vi "Define Mask.vi"(8 "error in (no error)":errorcluster, 11 "FPGA Image":T3(plugin-control)=refnum) -> (0 "error out":errorcluster)   [LabVIEW 2013]
doc: "GUI for selecting a part type and starting a batch process\nPart types list is passed in from caller.\nReturns when Start or Cancel is pressed."
uses:
  Sectors/Number of Wing Sector.ctl
  Mask ROI FG Enum.ctl
  Mask ROI Cluster.ctl
  Common/File IO/INI/Read write mode.ctl
  Message Passing/MsgQ Loops enum.ctl
  System Status/Status FG Enum.ctl
  Common/State Machines/State Machine Lib.lvlib
  Common/GUI/GUI.lvlib
  <vilib>/vision/NI_Vision_Development_Module.lvlib
  Image Processing.lvlib
  Message Passing/Main MsgQ.lvlib
panel:
  in  "Calculate BG":bool
  in  "Load Current Mask":bool
  out "Right ROI":T1 {"Contours"."Type" items=["No Selection", "Point", "Line", "Rectangle", "Oval", "Polygon", "Freehand Region", "Annulus", "Unused2", "Unused3", "Broken Line", "Freehand Line", "Rotated Rectangle"]}
  out "Left ROI":T1 {"Contours"."Type" items=["No Selection", "Point", "Line", "Rectangle", "Oval", "Polygon", "Freehand Region", "Annulus", "Unused2", "Unused3", "Broken Line", "Freehand Line", "Rotated Rectangle"]}
  out "[Avg BG]":dbl[](array[numeric])
  in  "NumWingSectors":T2=1 items=["1"=1, "2"=2, "4"=4, "8"=8, "16"=16]
  out "State":string
  in  "Exit":bool
  in  "Save Mask":bool
  out "combo mask":T3(plugin-control)
  out "right mask":T3(plugin-control)
  out "right masked image":T3(plugin-control)
  out "right annulus":T4={"Center X"=929, "Center Y"=663, "Inner Radius"=200, "Outer Radius"=405, "Start Angle"=90.0, "End Angle"=180.0} {"End Angle" format="%.2f"; "Start Angle" format="%.2f"; "Center X" scale=0.0..1024.0}
  out "left mask":T3(plugin-control)
  out "left masked image":T3(plugin-control)
  out "left annulus":T4={"Center X"=929, "Center Y"=663, "Inner Radius"=200, "Outer Radius"=405, "Start Angle"=90.0, "End Angle"=180.0} {"End Angle" format="%.2f"; "Start Angle" format="%.2f"; "Center X" scale=0.0..1024.0}
  in  "Accept Threshold":bool
  out "Processed Image":T3(plugin-control)
  in  "Threshold Range":cluster{"Lower value":dbl, "Upper value":dbl}={"Lower value"=106.82432432432432, "Upper value"=255.0} {"Upper value" min=0.0 max=255.0 scale=0.0..255.0; "Lower value" min=0.0 max=255.0}
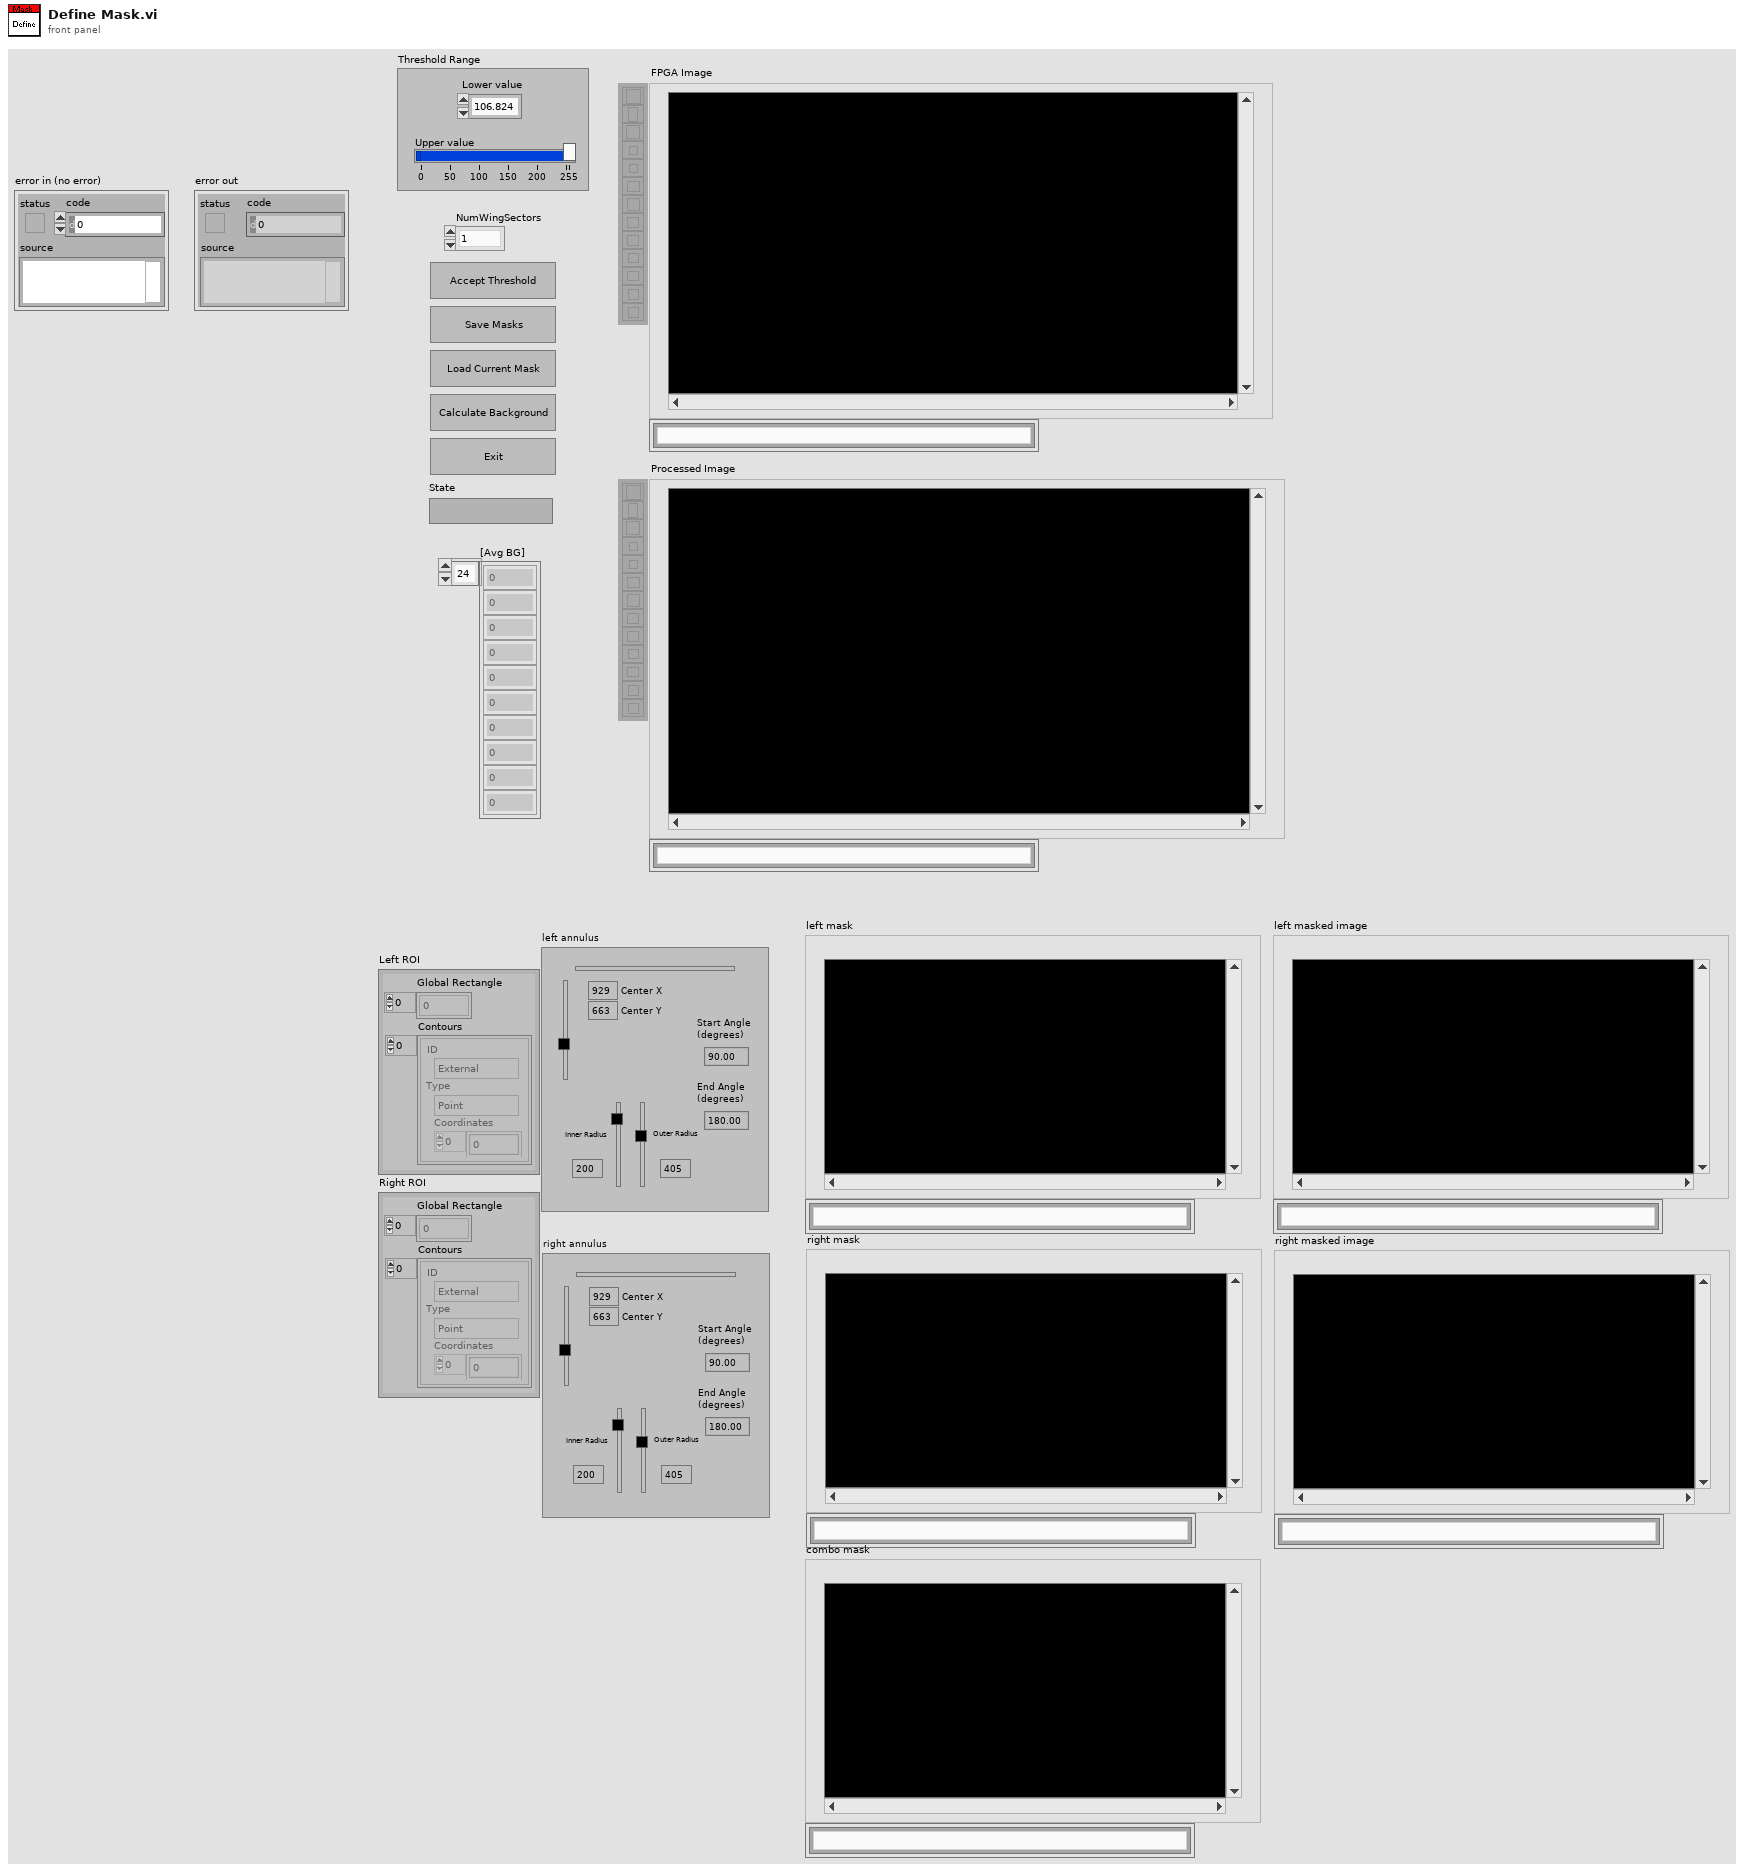
[diagram p1: front panel]
types:
  T1 = typedef "ROI Descriptor" = cluster{"Global Rectangle":i32[], "Contours":cluster{"ID":enum32{"External", "Internal"}, "Type":u32, "Coordinates":i32[]}[]}
  T2 = typedef "Number of Wing Sector.ctl" = u8
  T3 = typedef "IMAQ Image.ctl" = refnum<image>
  T4 = typedef "IMAQ Circle" = cluster{"Center X":i32, "Center Y":i32, "Inner Radius":i32, "Outer Radius":i32, "Start Angle":dbl, "End Angle":dbl}
  T5 = typedef "State Machine Lib.lvlib/STATE cluster.ctl" = cluster{"State":string, "Parameters":variant}
  T6 = typedef "Mask ROI FG Enum.ctl" = enum16{"Read", "Write", "Enable Background", "Disable Background"}
  T7 = typedef "Main MsgQ.lvlib/MsgQ Loops enum.ctl" = enum16{"User Interface", "Image Acq"}
  T8 = typedef "Read write mode.ctl" = enum16{"Read", "Write"}
  T9 = typedef "Mask ROI Cluster.ctl" = cluster{"left annulus":T4, "right annulus":T4, "Threshold Range":cluster{"Lower value":dbl, "Upper value":dbl}, "[Avg BG]":u8[], "Number of Sectors":u8, "Left ROI":T1, "Right ROI":T1, "Left Start Angle Duty Cycle":fxp<+,8,0>, "Left End Angle Duty Cycle":fxp<+,8,0>, "Right End Angle Duty Cycle":fxp<+,8,0>, "Right Start Angle Duty Cycle":fxp<+,8,0>, "[Sector ROIs]":T1[]}
  T10 = typedef "Status FG Enum.ctl" = enum16{"Reset", "Read", "Write"}
  T11 = typedef "Sector Parameter Cluster.ctl" = cluster{"Start Angle":fxp<+/-,17,2>, "End Angle":fxp<+/-,17,2>, "Inner Radius":u16, "Outter Radius":u16, "Hinge X":u16, "Hinge Y":u16, "NumWingSectors":u8}
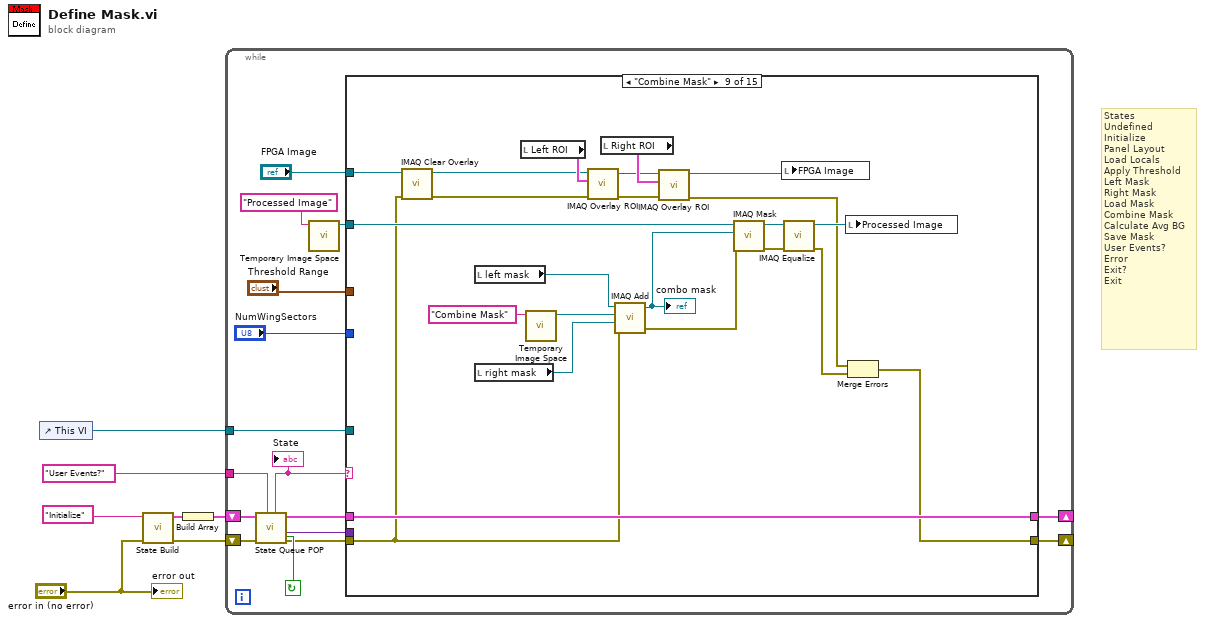
[diagram p0: block diagram]
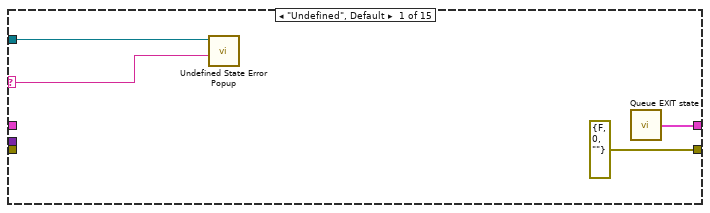
[diagram p2: hidden frame]
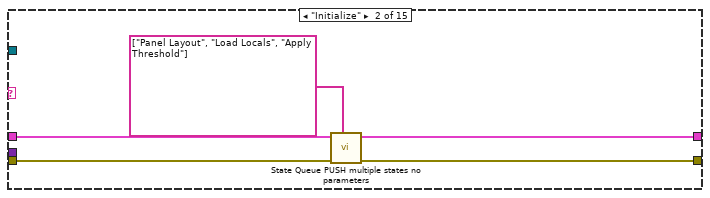
[diagram p3: hidden frame]
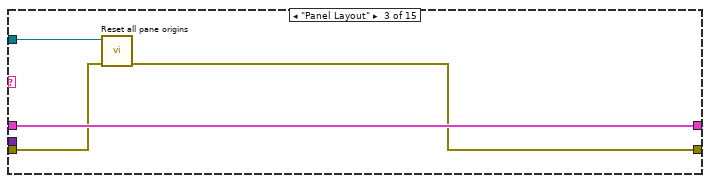
[diagram p4: hidden frame]
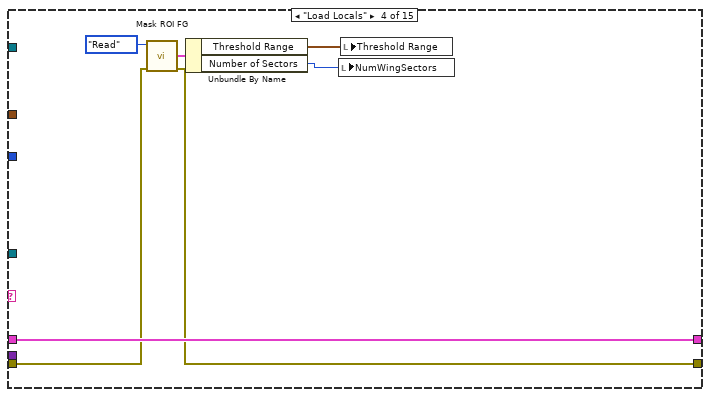
[diagram p5: hidden frame]
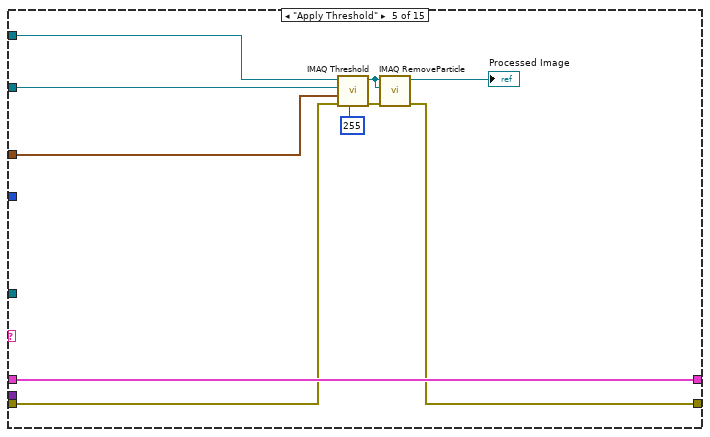
[diagram p6: hidden frame]
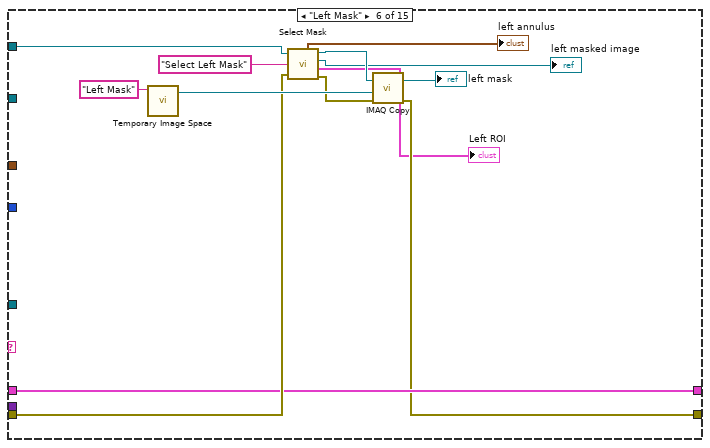
[diagram p7: hidden frame]
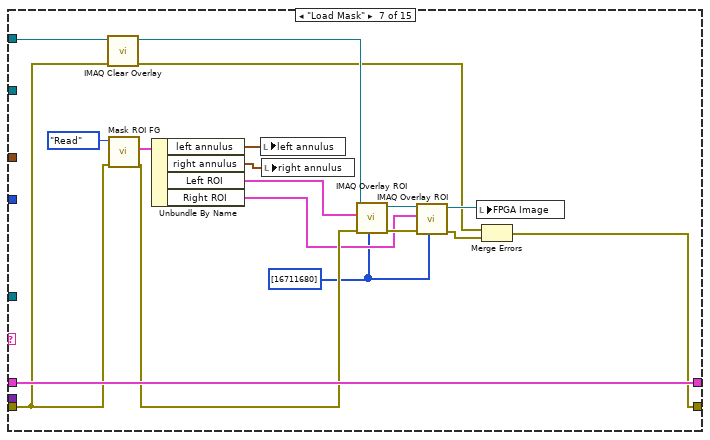
[diagram p8: hidden frame]
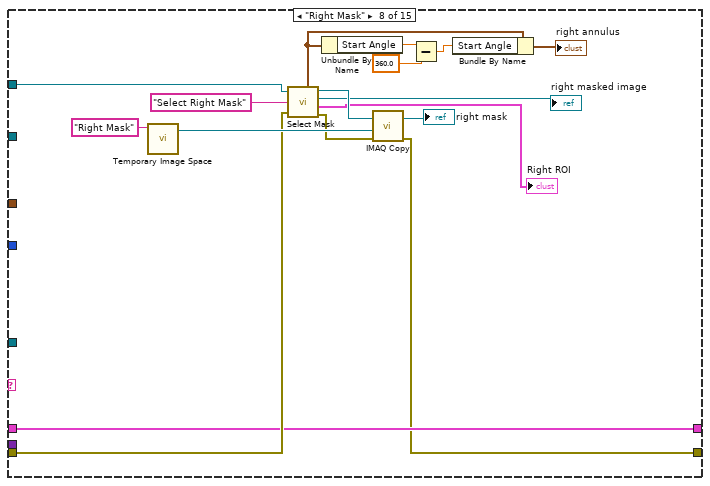
[diagram p9: hidden frame]
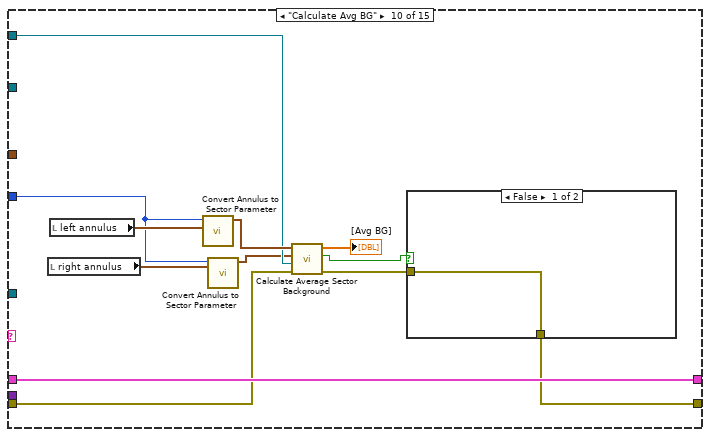
[diagram p10: hidden frame]
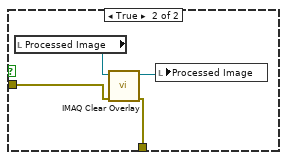
[diagram p11: hidden frame]
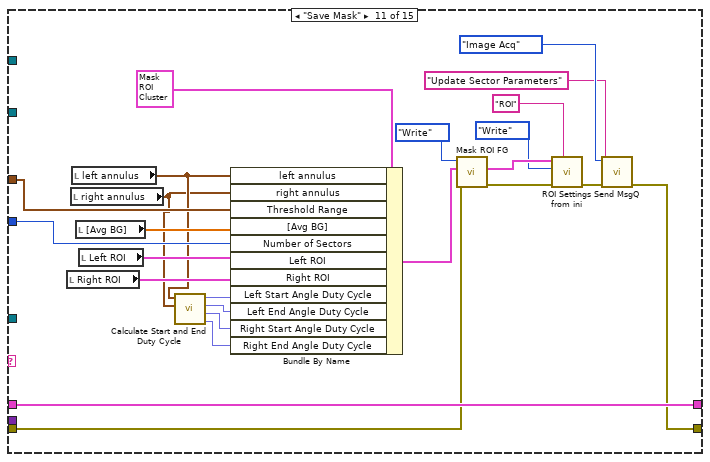
[diagram p12: hidden frame]
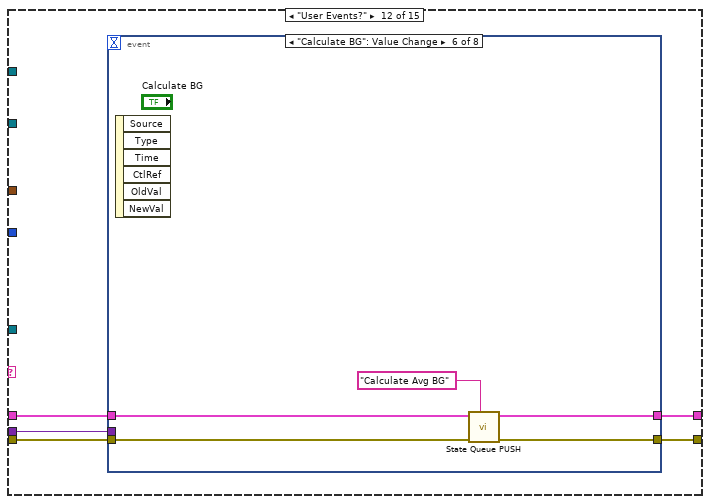
[diagram p13: hidden frame]
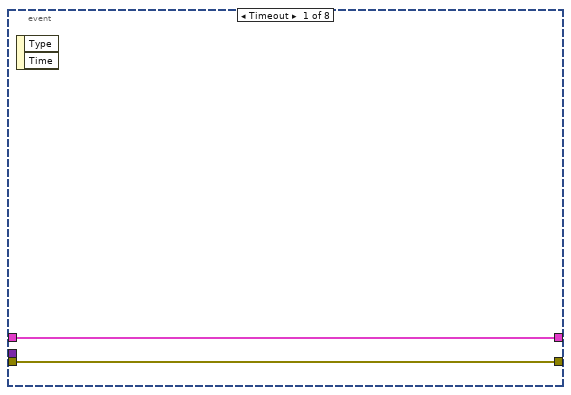
[diagram p14: hidden frame]
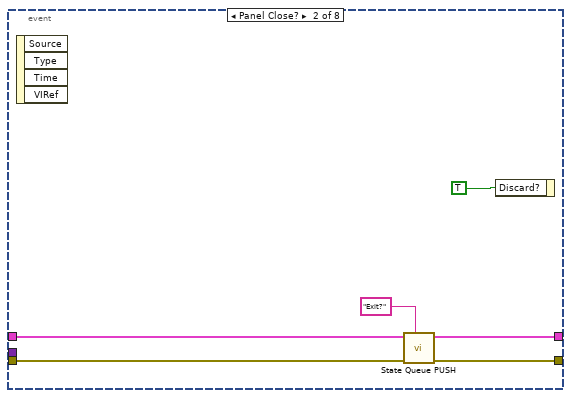
[diagram p15: hidden frame]
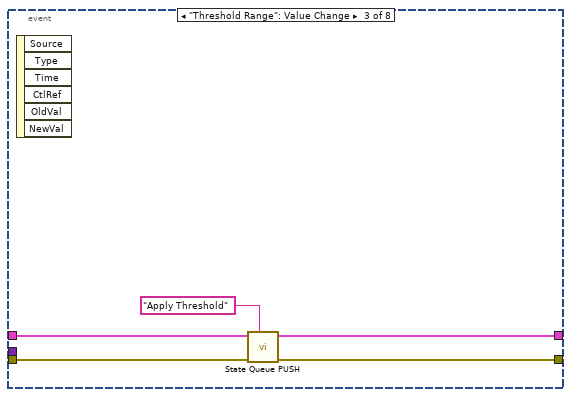
[diagram p16: hidden frame]
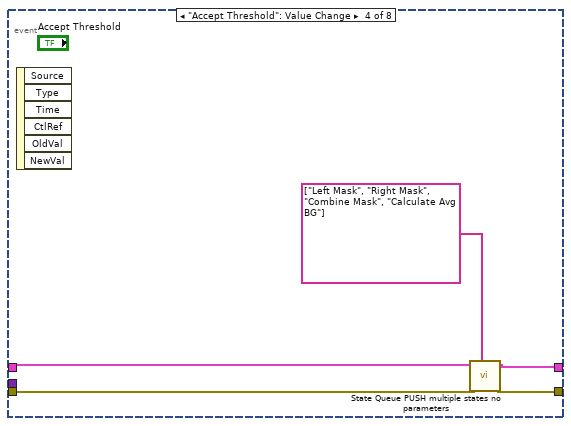
[diagram p17: hidden frame]
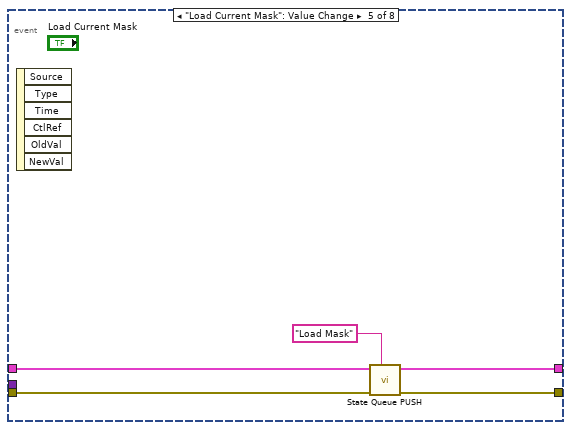
[diagram p18: hidden frame]
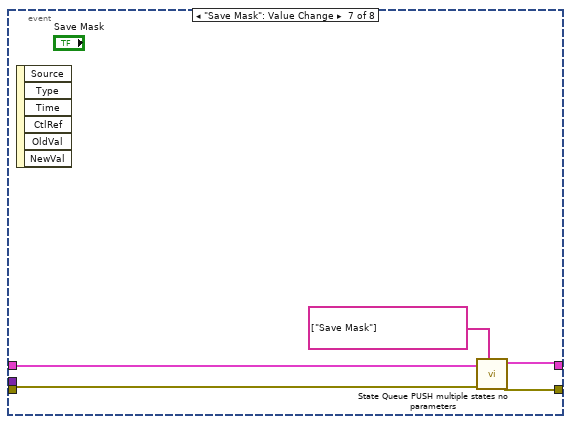
[diagram p19: hidden frame]
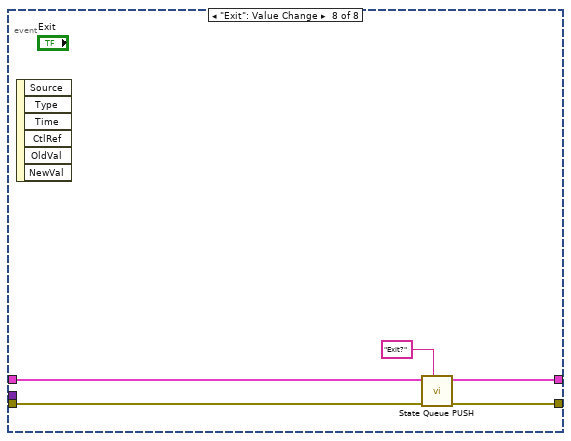
[diagram p20: hidden frame]
diagram:
  # "States\nUndefined\nInitialize\nPanel Layout\nLoad Locals\nApply Threshold\nLeft Mask\nRight Mask\nLoad Mask\nCombine Mask\nCalculate Avg BG\nSave Mask\nUser Events?\nError\nExit?\nExit"
  n1 = control-ref of="This VI"() -> (w6:refnum<vi>)
  n2 = call "State Build.vi"("error in (no error)"="error in (no error)", "State"="Initialize") -> ("error out"=w3:errorcluster, "State Out"=w4:T5)  [unwired: 8 in]
  n3 = Build Array(w4) -> (w5:T5[])
  n4 = while {
    shift-right: [w14] -> _
    shift-left: w3 -> [w22]
    shift-right: [w13] -> _
    shift-left: w5 -> [w20]
    tunnel: "User Events?" ("Default state") -> [w21]
    tunnel: w6 -> [w16]
    stop <- w23 continue-if-true
    n5 = call "State Queue POP.vi"("Default state"=w21, "error in (no error)"=w22, "State que in"=w20) -> ("error out"=w19:errorcluster, "Parameters"=w15:variant, "State que out"=w18:T5[], "Not Exit?"=w23:bool, "State case out"=w17:string)  [unwired: 4 out]
    "State" <- w17
    n6 = call "Temporary Image Space.vi"("Image Name"="Processed Image") -> ("Image Out"=w10:T3)  [unwired: 10 in]
    n7 = case shown="\"Combine Mask\"" w17 {
      selector: w17 -> [w24 _ _ _ _ _ _ _ _ _ _ _ _ _ _]
      tunnel: w19 -> [_ w30 w34 w42 w48 w59 w72 w94 w109 w135 w160 w169 w209 w223 w226]
      tunnel: w18 -> [_ w32 w36 w43 w49 w58 w83 w93 w114 w136 w165 w170 _ w217 w228]
      tunnel: w16 -> [w25 _ w35 _ _ _ _ _ _ _ _ _ _ _ _]
      tunnel: w15 -> [_ _ _ _ _ _ _ _ _ _ _ w168 _ _ _]
      tunnel: [errorcluster {"status"=FALSE, "code"=0, "source"=""} ("error out") w31 w33 w37 w47 w57 w67 w92 w102 w126 w150 w167 errorcluster {"status"=FALSE, "code"=0, "source"=""} ("error out") w223 w224] -> w14
      tunnel: [w27 w28 w36 w43 w49 w58 w83 w93 w114 w136 w165 w166 w214 w216 w228] -> w13
      tunnel: "Threshold Range" -> [_ _ _ _ w46 _ _ _ _ _ w162 _ _ _ _]
      tunnel: "FPGA Image" -> [_ _ _ _ w45 w60 w73 w95 w110 w132 _ _ _ _ w227]
      tunnel: w10 -> [_ _ _ _ w44 _ _ _ w117 _ _ _ _ _ _]
      tunnel: "NumWingSectors" -> [_ _ _ _ _ _ _ _ _ w130 w158 _ _ _ _]
      frame "Undefined", Default {
        n8 = call "Undefined State Error Popup.vi"("String"=w24, "This VI (Caller if unwired)"=w25) -> ()  [unwired: 10 out]
        n9 = call "Queue EXIT state.vi"() -> ("Exit State Q"=w27:T5[])  [unwired: 1 in]
      }
      frame "Initialize" {
        n10 = call "State Queue PUSH multiple states no parameters.vi"("States to queue"=string[] ["Panel Layout", "Load Locals", "Apply Threshold"], "error in (no error)"=w30, "State que in"=w32) -> ("error out"=w31:errorcluster, "State que out"=w28:T5[])  [unwired: 1 in, 6 out]
      }
      frame "Panel Layout" {
        n11 = call "Reset all pane origins.vi"("error in (no error"=w34, "Vi Ref In"=w35) -> ("error out"=w33:errorcluster)  [unwired: 9 out]
      }
      frame "Load Locals" {
        n12 = call "Mask ROI FG.vi"("error in (no error)"=w42, "Operation"=Mask_ROI_FG_Enum."Read") -> ("error out"=w37:errorcluster, "Mask ROI Out"=w40:T9)  [unwired: 8 in]
        n13 = Unbundle By Name(w40) -> ("Threshold Range"=w39:cluster{"Lower value":dbl, "Upper value":dbl}, "Number of Sectors"=w38:u8)
        n14 = local write "NumWingSectors"(w38) -> ()
        n15 = local write "Threshold Range"(w39) -> ()
      }
      frame "Apply Threshold" {
        n16 = call "IMAQ Threshold"("Replace Value"=u8 255, "error in (no error)"=w48, "Range"=w46, "Image Dst"=w44, "Image Src"=w45) -> ("error out"=w51:errorcluster, "Image Dst Out"=w53:T3)  [unwired: 1 in, 4 out]
        n17 = call "IMAQ RemoveParticle"("error in (no error)"=w51, "Image Dst"=w53, "Image Src"=w53) -> ("error out"=w47:errorcluster, "Image Dst Out"=→"Processed Image":T3)  [unwired: 4 in, 3 out]
      }
      frame "Left Mask" {
        n18 = call "Temporary Image Space.vi"("Image Name"="Left Mask") -> ("Image Out"=w61:T3)  [unwired: 10 in]
        n19 = call "Select Mask.vi"("error in"=w59, "Prompt"="Select Left Mask", "Read \nImage"=w60) -> ("error out"=w56:errorcluster, "ROI Descriptor Out"=→"Left ROI":T1, "Masked \nImage"=→"left masked image":T3, "Annulus"=→"left annulus":T4, "mask"=w64:T3)  [unwired: 1 out]
        n20 = call "IMAQ Copy"("error in (no error)"=w56, "Image Dst"=w61, "Image Src"=w64) -> ("error out"=w57:errorcluster, "Image Dst Out"=→"left mask":T3)  [unwired: 3 in]
      }
      frame "Load Mask" {
        w70 = u32[] [16711680] ("Colors (Green)")
        n21 = call "IMAQ Clear Overlay"("error in (no error)"=w72, "Image"=w73) -> ("error out"=w69:errorcluster, "Image Out"=w71:T3)  [unwired: 8 in]
        n22 = call "Mask ROI FG.vi"("error in (no error)"=w72, "Operation"=Mask_ROI_FG_Enum."Read") -> ("error out"=w76:errorcluster, "Mask ROI Out"=w82:T9)  [unwired: 8 in]
        n23 = Unbundle By Name(w82) -> ("left annulus"=w81:T4, "right annulus"=w80:T4, "Left ROI"=w75:T1, "Right ROI"=w74:T1)
        n24 = local write "left annulus"(w81) -> ()
        n25 = local write "right annulus"(w80) -> ()
        n26 = call "IMAQ Overlay ROI"("Colors (Green)"=w70, "error in (no error)"=w76, "ROI Descriptor"=w75, "Image"=w71) -> ("error out"=w77:errorcluster, "Image Out"=w79:T3)  [unwired: 6 in]
        n27 = call "IMAQ Overlay ROI"("Colors (Green)"=w70, "error in (no error)"=w77, "ROI Descriptor"=w74, "Image"=w79) -> ("error out"=w68:errorcluster, "Image Out"=w78:T3)  [unwired: 6 in]
        n28 = local write "FPGA Image"(w78) -> ()
        n29 = Merge Errors(w69, w68) -> (w67:errorcluster)
      }
      frame "Right Mask" {
        n30 = call "Temporary Image Space.vi"("Image Name"="Right Mask") -> ("Image Out"=w96:T3)  [unwired: 10 in]
        n31 = call "Select Mask.vi"("error in"=w94, "Prompt"="Select Right Mask", "Read \nImage"=w95) -> ("error out"=w91:errorcluster, "ROI Descriptor Out"=→"Right ROI":T1, "Masked \nImage"=→"right masked image":T3, "Annulus"=w85:T4, "mask"=w99:T3)  [unwired: 1 out]
        n32 = Unbundle By Name(w85) -> ("Start Angle"=w90:dbl)
        n33 = call "IMAQ Copy"("error in (no error)"=w91, "Image Dst"=w96, "Image Src"=w99) -> ("error out"=w92:errorcluster, "Image Dst Out"=→"right mask":T3)  [unwired: 3 in]
        n34 = Subtract(x=w90, y=360.0) -> (x-y=w88:dbl)
        n35 = Bundle By Name(cluster=w85, "Start Angle"=w88) -> (→"right annulus":T4)
      }
      frame "Combine Mask" {
        n36 = call "IMAQ Clear Overlay"("error in (no error)"=w109, "Image"=w110) -> ("error out"=w108:errorcluster, "Image Out"=w107:T3)  [unwired: 8 in]
        n37 = local read "left mask"() -> (w119:T3)
        n38 = local read "right mask"() -> (w118:T3)
        n39 = local read "Left ROI"() -> (w113:T1)
        n40 = call "Temporary Image Space.vi"("Image Name"="Combine Mask") -> ("Image Out"=w121:T3)  [unwired: 10 in]
        n41 = call "IMAQ Overlay ROI"("error in (no error)"=w108, "ROI Descriptor"=w113, "Image"=w107) -> ("error out"=w106:errorcluster, "Image Out"=w105:T3)  [unwired: 7 in]
        n42 = local read "Right ROI"() -> (w112:T1)
        n43 = call "IMAQ Add"("Image Src A"=w119, "Image Dst"=w121, "Image Src B"=w118, "error in (no error)"=w109) -> ("Image Dst Out"=w122:T3, "error out"=w115:errorcluster)  [unwired: 3 in]
        "combo mask" <- w122
        n44 = call "IMAQ Overlay ROI"("error in (no error)"=w106, "ROI Descriptor"=w112, "Image"=w105) -> ("error out"=w104:errorcluster, "Image Out"=w111:T3)  [unwired: 7 in]
        n45 = call "IMAQ Mask"("error in (no error)"=w115, "Image Mask"=w122, "Image Src"=w117) -> ("error out"=w123:errorcluster, "Image Dst Out"=w124:T3)  [unwired: 1 in, 1 out]
        n46 = local write "FPGA Image"(w111) -> ()
        n47 = call "IMAQ Equalize"("error in (no error)"=w123, "Image Src"=w124) -> ("error out"=w103:errorcluster, "Image Dst Out"=w116:T3)  [unwired: 4 in, 4 out]
        n48 = local write "Processed Image"(w116) -> ()
        n49 = Merge Errors(w104, w103) -> (w102:errorcluster)
      }
      frame "Calculate Avg BG" {
        n50 = local read "right annulus"() -> (w129:T4)
        n51 = local read "left annulus"() -> (w134:T4)
        n52 = call "Convert Annulus to Sector Parameter.vi"("Annulus"=w134, "NumWingSectors"=w130) -> ("Sector Parameter"=w133:T11)  [unwired: 9 in]
        n53 = call "Convert Annulus to Sector Parameter.vi"("Annulus"=w129, "NumWingSectors"=w130) -> ("Sector Parameter"=w128:T11)  [unwired: 9 in]
        n54 = call "Calculate Average Sector Background.vi"("error in (no error)"=w135, "Image"=w132, "Right Sector Parameters"=w128, "Left Sector Parameters"=w133) -> ("error out"=w127:errorcluster, "Canceled?"=w125:bool, "[Avg BG]"=→"[Avg BG]":dbl[])  [unwired: 5 in]
        n55 = case shown="False" w125 {
          tunnel: w127 -> [w137 w140]
          tunnel: [w137 w139] -> w126
          frame False {
          }
          frame True {
            n56 = local read "Processed Image"() -> (w141:T3)
            n57 = call "IMAQ Clear Overlay"("error in (no error)"=w140, "Image"=w141) -> ("error out"=w139:errorcluster, "Image Out"=w138:T3)  [unwired: 8 in]
            n58 = local write "Processed Image"(w138) -> ()
          }
        }
      }
      frame "Save Mask" {
        n59 = local read "Right ROI"() -> (w148:T1)
        n60 = local read "right annulus"() -> (w146:T4)
        n61 = local read "left annulus"() -> (w147:T4)
        n62 = local read "[Avg BG]"() -> (w159:dbl[])
        n63 = local read "Left ROI"() -> (w149:T1)
        n64 = call "Calculate Start and End Duty Cycle.vi"("right annulus"=w146, "left annulus"=w147) -> ("Right End Angle Duty Cycle"=w142:fxp<+,8,0>, "Right Start Angle Duty Cycle"=w143:fxp<+,8,0>, "Left End Angle Duty Cycle"=w144:fxp<+,8,0>, "Left Start Angle Duty Cycle"=w145:fxp<+,8,0>)  [unwired: 6 in]
        n65 = Bundle By Name(cluster=T9 {"left annulus"={"Center X"=929, "Center Y"=663, "Inner Radius"=200, "Outer Radius"=405, "Start Angle"=90.0, "End Angle"=180.0}, "right annulus"={"Center X"=929, "Center Y"=663, "Inner Radius"=200, "Outer Radius"=405, "Start Angle"=90.0, "End Angle"=180.0}, "Threshold Range"={"Lower value"=106.82432432432432, "Upper value"=255.0}, "[Avg BG]"=[], "Number of Sectors"=0, "Left ROI"={"Global Rectangle"=[], "Contours"=[]}, "Right ROI"={"Global Rectangle"=[], "Contours"=[]}, "Left Start Angle Duty Cycle"=0.0, "Left End Angle Duty Cycle"=0.0, "Right End Angle Duty Cycle"=0.0, "Right Start Angle Duty Cycle"=0.0, "[Sector ROIs]"=[]} ("Mask ROI In"), "left annulus"=w147, "right annulus"=w146, "Threshold Range"=w162, "[Avg BG]"=w159, "Number of Sectors"=w158, "Left ROI"=w149, "Right ROI"=w148, "Left Start Angle Duty Cycle"=w145, "Left End Angle Duty Cycle"=w144, "Right Start Angle Duty Cycle"=w143, "Right End Angle Duty Cycle"=w142) -> (w161:T9)
        n66 = call "Mask ROI FG.vi"("error in (no error)"=w160, "Mask ROI In"=w161, "Operation"=Mask_ROI_FG_Enum."Write") -> ("error out"=w155:errorcluster, "Mask ROI Out"=w157:T9)  [unwired: 7 in]
        n67 = call "ROI Settings from ini.vi"("Section"="ROI", "error in (no error)"=w155, "Operation"=Read_write_mode."Write", "Mask ROI In"=w157) -> ("error out"=w151:errorcluster)  [unwired: 5 in, 2 out]
        n68 = call "Send MsgQ.vi"("error in (no error)"=w151, "Message String"="Update Sector Parameters", "Send to MsgQ"=MsgQ_Loops_enum."Image Acq") -> ("error out"=w150:errorcluster)  [unwired: 8 in]
      }
      frame "User Events?" {
        n69 = event shown="[5] \"Calculate BG\": Value Change" {
          selector: _ -> [_ _ _ _ _ _ _ _]
          dyn-events: _ -> [_ _ _ _ _ _ _ _]
          timeout: _ -> [_ _ _ _ _ _ _ _]
          tunnel: w170 -> [w171 w177 w183 w186 w192 w197 w202 w205]
          tunnel: w169 -> [w172 w176 w182 w184 w189 w194 w199 w206]
          tunnel: w168 -> [_ _ _ _ _ _ _ _]
          tunnel: [w172 w174 w180 w187 w190 w195 w200 w207] -> w167
          tunnel: [w171 w175 w181 w188 w191 w196 w201 w208] -> w166
          event Timeout {
            n70 = event-data() -> ()  [unwired: 3 out]
          }
          event Panel Close? {
            n71 = event-data() -> ()  [unwired: 5 out]
            n72 = call "State Queue PUSH.vi"("State case"="Exit?", "error in (no error)"=w176, "State que in"=w177) -> ("error out"=w174:errorcluster, "State que out"=w175:T5[])  [unwired: 2 in, 5 out]
            n73 = event-data("Discard?"=TRUE) -> ()  [unwired: 1 in, 1 out]
          }
          event "Threshold Range": Value Change {
            n74 = event-data() -> ()  [unwired: 7 out]
            n75 = call "State Queue PUSH.vi"("State case"="Apply Threshold", "error in (no error)"=w182, "State que in"=w183) -> ("error out"=w180:errorcluster, "State que out"=w181:T5[])  [unwired: 2 in, 5 out]
          }
          event "Accept Threshold": Value Change {
            n76 = event-data() -> ()  [unwired: 7 out]
            n77 = call "State Queue PUSH multiple states no parameters.vi"("States to queue"=string[] ["Left Mask", "Right Mask", "Combine Mask", "Calculate Avg BG"], "error in (no error)"=w184, "State que in"=w186) -> ("error out"=w187:errorcluster, "State que out"=w188:T5[])  [unwired: 7 in]
          }
          event "Load Current Mask": Value Change {
            n78 = event-data() -> ()  [unwired: 7 out]
            n79 = call "State Queue PUSH.vi"("State case"="Load Mask", "error in (no error)"=w189, "State que in"=w192) -> ("error out"=w190:errorcluster, "State que out"=w191:T5[])  [unwired: 2 in, 5 out]
          }
          event "Calculate BG": Value Change {
            n80 = event-data() -> ()  [unwired: 7 out]
            n81 = call "State Queue PUSH.vi"("State case"="Calculate Avg BG", "error in (no error)"=w194, "State que in"=w197) -> ("error out"=w195:errorcluster, "State que out"=w196:T5[])  [unwired: 2 in, 5 out]
          }
          event "Save Mask": Value Change {
            n82 = event-data() -> ()  [unwired: 7 out]
            n83 = call "State Queue PUSH multiple states no parameters.vi"("States to queue"=string[] ["Save Mask"], "error in (no error)"=w199, "State que in"=w202) -> ("error out"=w200:errorcluster, "State que out"=w201:T5[])  [unwired: 7 in]
          }
          event "Exit": Value Change {
            n84 = event-data() -> ()  [unwired: 7 out]
            n85 = call "State Queue PUSH.vi"("State case"="Exit?", "error in (no error)"=w206, "State que in"=w205) -> ("error out"=w207:errorcluster, "State que out"=w208:T5[])  [unwired: 7 in]
          }
        }
      }
      frame "Error" {
        # "DEFAULT IS \nTO CLEAR ERROR\nAND EXIT"
        n86 = Unbundle By Name(w209) -> ("source"=w212:string)
        n87 = Concatenate Strings("Error: " ("string"), w212) -> (w211:string)
        n88 = call "Status FG.vi"("Status In"=w211, "Operation"=Status_FG_Enum."Write") -> ()  [unwired: 8 in, 2 out]
        n89 = call <vilib>:"Clear Errors.vi"("error in (no error)"=w209) -> ()  [unwired: 7 out]
        n90 = call "Queue EXIT state.vi"() -> ("Exit State Q"=w214:T5[])  [unwired: 1 in]
      }
      frame "Exit?" {
        n91 = Two Button Dialog(message="Exit?", 1:"No" ("F button name (\"Cancel\")"), 2:"Yes" ("T button name (\"OK\")")) -> (T button?=w219:bool)
        n92 = call "Queue EXIT state.vi"() -> ("Exit State Q"=w218:T5[])  [unwired: 1 in]
        n93 = Select(t=w218, s=w219, f=w217) -> (s? t:f=w216:T5[])
      }
      frame "Exit" {
        n94 = call "IMAQ Clear Overlay"("error in (no error)"=w226, "Image"=w227) -> ("error out"=w225:errorcluster)  [unwired: 8 in, 1 out]
        n95 = call <vilib>:"Clear Errors.vi"("error in (no error)"=w225) -> ("error out"=w224:errorcluster)  [unwired: 6 in]
      }
    }
  }
  "error out" <- "error in (no error)"
